vi "Signal Manipulation.vi"(4 "Center":dbl[](array[numeric]), 5 "Tank Pressure":dbl[](array[numeric]), 6 "Post":dbl[](array[numeric]), 7 "Chamber Pressure":dbl[](array[numeric]), 8 "Pre":dbl[](array[numeric]), 9 "Injector":dbl[](array[numeric]), 10 "Thrust":dbl[](array[numeric]), 11 "Tank Mass":dbl[](array[numeric])) -> (3 "Dynamic Data":dynamicdata(waveform))   [LabVIEW 2021]
uses:
  <vilib>/ptbypt/NI_PtbyPt.lvlib
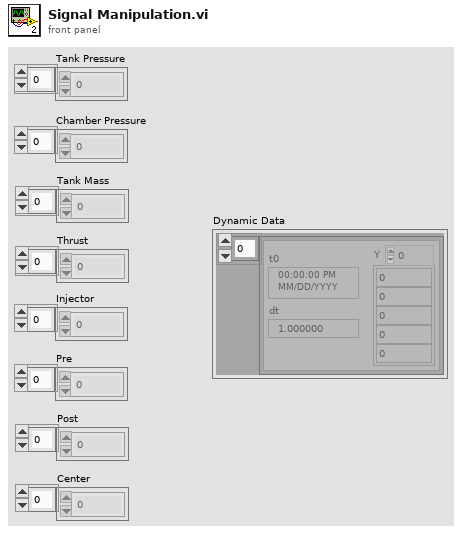
[diagram p1: front panel]
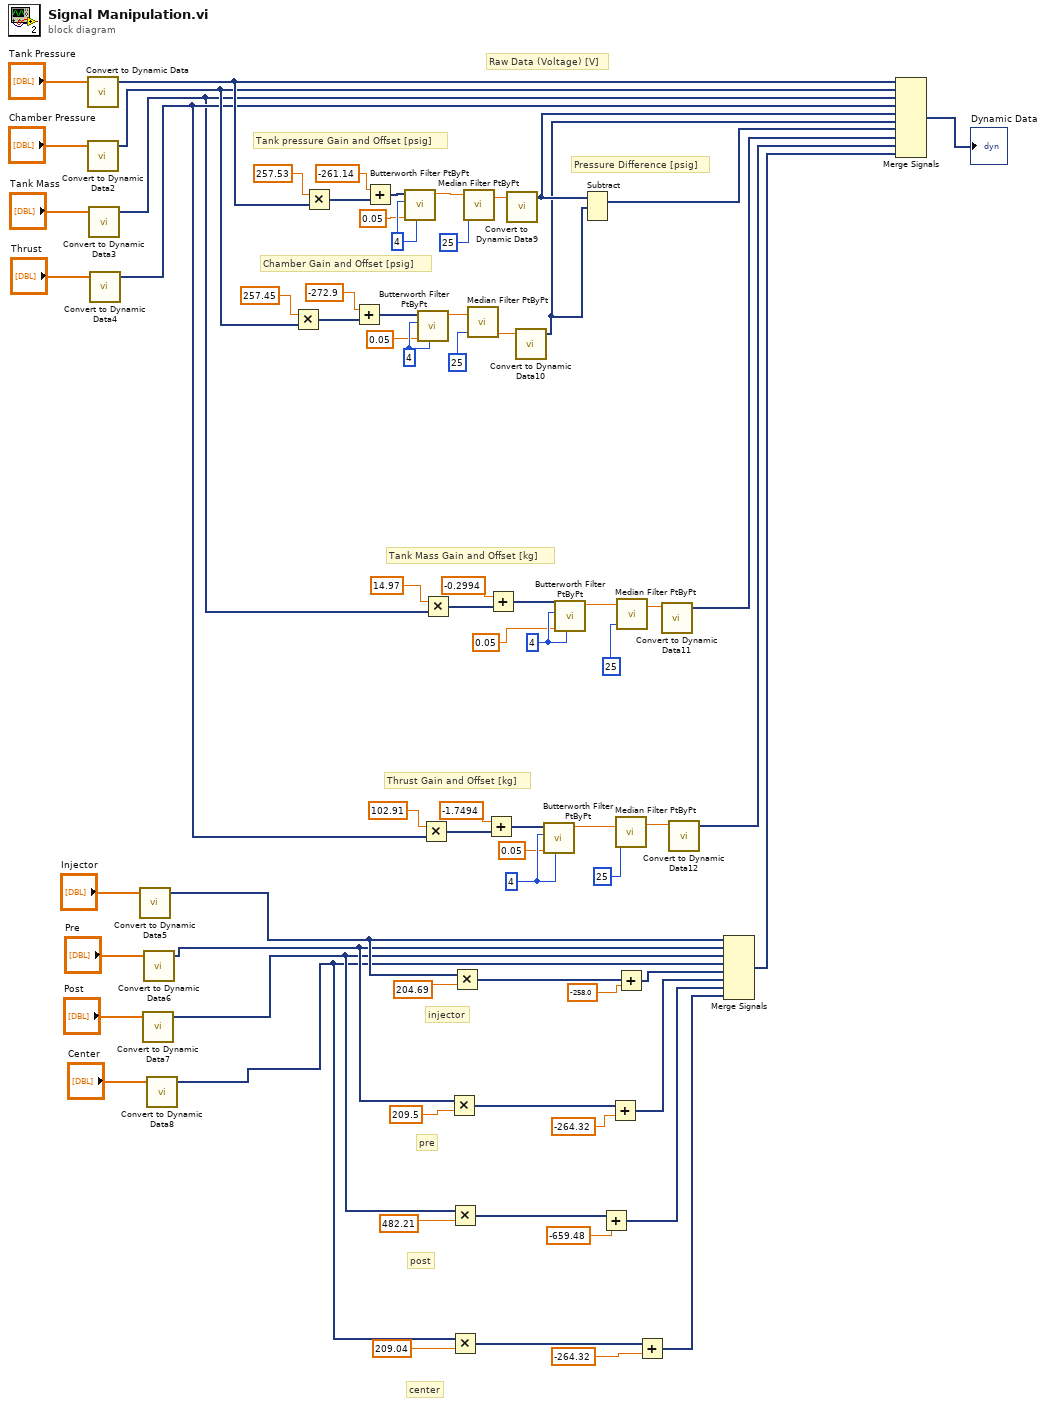
[diagram p0: block diagram]
diagram:
  w48 = 4
  w49 = 4
  w50 = 4
  w51 = 4
  # "center"
  # "post"
  # "pre"
  # "injector"
  # "Thrust Gain and Offset [kg]"
  # "Raw Data (Voltage) [V]"
  # "Pressure Difference [psig]"
  # "Tank Mass Gain and Offset [kg]"
  # "Chamber Gain and Offset [psig]"
  # "Tank pressure Gain and Offset [psig]"
  n1 = call "Convert to Dynamic Data"("Array"="Tank Pressure") -> ("Dynamic Data Type"=w23:dynamicdata)  [unwired: 3 in]
  n2 = call "Convert to Dynamic Data2"("Array"="Chamber Pressure") -> ("Dynamic Data Type"=w15:dynamicdata)  [unwired: 3 in]
  n3 = call "Convert to Dynamic Data3"("Array"="Tank Mass") -> ("Dynamic Data Type"=w13:dynamicdata)  [unwired: 3 in]
  n4 = call "Convert to Dynamic Data4"("Array"="Thrust") -> ("Dynamic Data Type"=w14:dynamicdata)  [unwired: 3 in]
  n5 = call "Convert to Dynamic Data5"("Array"="Injector") -> ("Dynamic Data Type"=w12:dynamicdata)  [unwired: 3 in]
  n6 = call "Convert to Dynamic Data7"("Array"="Post") -> ("Dynamic Data Type"=w10:dynamicdata)  [unwired: 3 in]
  n7 = call "Convert to Dynamic Data6"("Array"="Pre") -> ("Dynamic Data Type"=w11:dynamicdata)  [unwired: 3 in]
  n8 = call "Convert to Dynamic Data8"("Array"="Center") -> ("Dynamic Data Type"=w9:dynamicdata)  [unwired: 3 in]
  n9 = Multiply(x=257.45, y=w15) -> (x*y=w67:dynamicdata)
  n10 = Multiply(x=257.53, y=w23) -> (x*y=w66:dynamicdata)
  n11 = Add(x=-272.9, y=w67) -> (x+y=w61:dynamicdata)
  n12 = Add(x=-261.14, y=w66) -> (x+y=w25:dynamicdata)
  n13 = call <vilib>:"Butterworth Filter PtByPt.vi"("order"=w48, "low cutoff freq: fl"=0.05, "sampling freq: fs"=w48, "x"=w25) -> ("Filtered x"=w62:dbl)  [unwired: 5 in, 1 out]
  n14 = call <vilib>:"Butterworth Filter PtByPt.vi"("order"=w49, "low cutoff freq: fl"=0.05, "sampling freq: fs"=w49, "x"=w61) -> ("Filtered x"=w60:dbl)  [unwired: 5 in, 1 out]
  n15 = Multiply(x=102.91, y=w14) -> (x*y=w63:dynamicdata)
  n16 = Multiply(x=14.97, y=w13) -> (x*y=w68:dynamicdata)
  n17 = Multiply(x=w11, y=209.5) -> (x*y=w40:dynamicdata)
  n18 = Multiply(x=w10, y=482.21) -> (x*y=w41:dynamicdata)
  n19 = Multiply(x=w9, y=209.04) -> (x*y=w42:dynamicdata)
  n20 = Multiply(x=w12, y=204.69) -> (x*y=w31:dynamicdata)
  n21 = call <vilib>:"Median Filter PtByPt.vi"("rank"=25, "x"=w62) -> ("Filtered x"=w8:dbl)  [unwired: 2 in, 1 out]
  n22 = call <vilib>:"Median Filter PtByPt.vi"("rank"=25, "x"=w60) -> ("Filtered x"=w6:dbl)  [unwired: 2 in, 1 out]
  n23 = Add(x=-1.7494, y=w63) -> (x+y=w57:dynamicdata)
  n24 = Add(x=-0.2994, y=w68) -> (x+y=w59:dynamicdata)
  n25 = call "Convert to Dynamic Data9"("Double"=w8) -> ("Dynamic Data Type"=w7:dynamicdata)  [unwired: 3 in]
  n26 = call "Convert to Dynamic Data10"("Double"=w6) -> ("Dynamic Data Type"=w5:dynamicdata)  [unwired: 3 in]
  n27 = call <vilib>:"Butterworth Filter PtByPt.vi"("order"=w51, "low cutoff freq: fl"=0.05, "sampling freq: fs"=w51, "x"=w57) -> ("Filtered x"=w56:dbl)  [unwired: 5 in, 1 out]
  n28 = call <vilib>:"Butterworth Filter PtByPt.vi"("order"=w50, "low cutoff freq: fl"=0.05, "sampling freq: fs"=w50, "x"=w59) -> ("Filtered x"=w58:dbl)  [unwired: 5 in, 1 out]
  n29 = Subtract(1:w5, 2:w7) -> (0:w43:dynamicdata)  [unwired: 1 in, 1 out]
  n30 = Add(x=w41, y=-659.48) -> (x+y=w28:dynamicdata)
  n31 = Add(x=w40, y=-264.32) -> (x+y=w29:dynamicdata)
  n32 = call <vilib>:"Median Filter PtByPt.vi"("rank"=25, "x"=w56) -> ("Filtered x"=w4:dbl)  [unwired: 2 in, 1 out]
  n33 = Add(x=w31, y=-258.0) -> (x+y=w30:dynamicdata)
  n34 = call <vilib>:"Median Filter PtByPt.vi"("rank"=25, "x"=w58) -> ("Filtered x"=w2:dbl)  [unwired: 2 in, 1 out]
  n35 = Add(x=w42, y=-264.32) -> (x+y=w27:dynamicdata)
  n36 = call "Convert to Dynamic Data11"("Double"=w2) -> ("Dynamic Data Type"=w1:dynamicdata)  [unwired: 3 in]
  n37 = call "Convert to Dynamic Data12"("Double"=w4) -> ("Dynamic Data Type"=w3:dynamicdata)  [unwired: 3 in]
  n38 = Merge Signals(w12, w11, w10, w9, w30, w29, w28, w27) -> (w26:dynamicdata)
  n39 = Merge Signals(w23, w15, w13, w14, w7, w5, w43, w1, w3, w26) -> (→"Dynamic Data":dynamicdata)
